vi "PXIe4309GetRate.vi"(10 "Physical Channel\nEnable":bool[](array[boolean]), 11 "Physical Channels":tag[](array[tag])) -> (3 "Sampling Rate":dbl)   [LabVIEW 2020]
uses:
  c4962d46-b3fb-4968-a2a4-428a4d5ddc52.vi
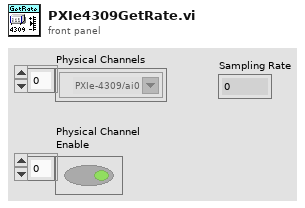
[diagram p1: front panel]
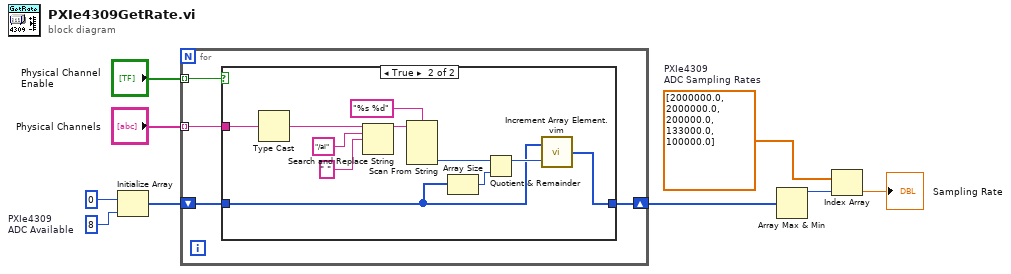
[diagram p0: block diagram]
diagram:
  w2 = dbl[] [2000000.0, 2000000.0, 200000.0, 133000.0, 100000.0]  # PXIe4309 ADC Sampling Rates
  w7 = 8  # PXIe4309 ADC Available
  n1 = Initialize Array(0 ("element"), w7) -> (w5:i32[])
  n2 = for {
    tunnel: "Physical Channels" -> [w13] mode=indexing
    tunnel: "Physical Channel\nEnable" -> [w12] mode=indexing
    shift-right: [w10] -> w3
    shift-left: w5 -> [w11]
    n3 = case shown="True" w12 {
      tunnel: w13 -> [_ w19]
      tunnel: w11 -> [w14 w16]
      tunnel: [w14 w15] -> w10
      frame False {
      }
      frame True {
        n4 = Type Cast(x=w19) -> (*(type *) &x=w21:string)  [unwired: 1 in]
        n5 = Search and Replace String(input string=w21, search string="/ai", replace string=" " ("replace string (\"\")")) -> (result string=w20:string)  [unwired: 5 in, 3 out]
        n6 = Scan From String(format string="%s %d", input string=w20) -> (output 2=w24:i32)  [unwired: 5 in, 3 out]
        n7 = Array Size(array=w16) -> (size(s)=w17:i32)
        n8 = Quotient & Remainder(x=w24, y=w17) -> (x-y*floor(x/y)=w18:i32)  [unwired: 1 out]
        n9 = call "Increment Array Element.vim"("index"=w18, "array in"=w16) -> ("array out"=w15:i32[])
      }
    }
  }
  n10 = Array Max & Min(array=w3) -> (max value=w4:i32)  [unwired: 3 out]
  n11 = Index Array(array=w2, index=w4) -> (element=→"Sampling Rate":dbl)
